vi "test.vi"() -> ()   [LabVIEW 2020, in "lvzstd.lvlib"]
uses:
  lvzstd.lvlib
panel:
  out "uncompressed data":string
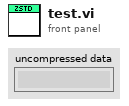
[diagram p1: front panel]
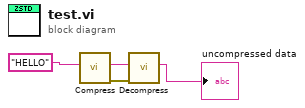
[diagram p0: block diagram]
diagram:
  n1 = call "Compress.vi"("data in"="HELLO") -> ("error out"=w3:errorcluster, "compressed data"=w2:string)  [unwired: 9 in]
  n2 = call "Decompress.vi"("error in (no error)"=w3, "compressed data"=w2) -> ("uncompressed data"=→"uncompressed data":string)  [unwired: 8 in, 1 out]
